vi "控制VI的显示方式.vi"() -> ()   [LabVIEW 2011]
panel:
  in  "方式":T1(ring)
  in  "stop":bool
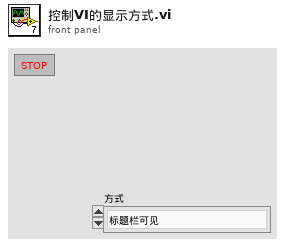
[diagram p1: front panel]
types:
  T1 = enum16{"标题栏可见", "标题栏不可见", "工具栏可见", "工具栏不可见", "菜单条可见", "菜单条不可见"}
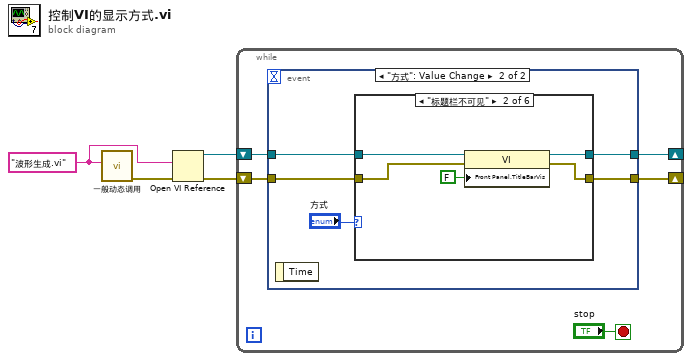
[diagram p0: block diagram]
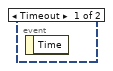
[diagram p2: hidden frame]
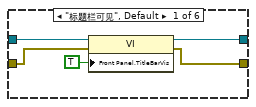
[diagram p3: hidden frame]
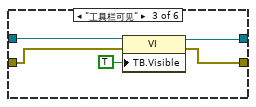
[diagram p4: hidden frame]
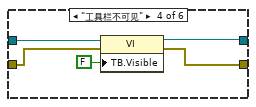
[diagram p5: hidden frame]
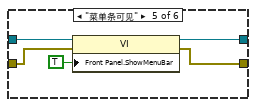
[diagram p6: hidden frame]
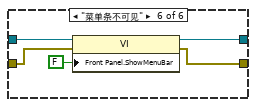
[diagram p7: hidden frame]
diagram:
  w3 = "波形生成.vi" ("name or relative path")
  n1 = call "一般动态调用.vi"("name or relative path"=w3) -> ("error out"=w4:errorcluster)  [unwired: 10 in]
  n2 = Open VI Reference(vi path=w3, error in (no error)=w4) -> (vi reference=w2:refnum<vi>, error out=w1:errorcluster)  [unwired: 4 in]
  n3 = while {
    shift-right: [w6] -> _
    shift-left: w2 -> [w8]
    shift-right: [w5] -> _
    shift-left: w1 -> [w7]
    stop <- "stop" stop-if-true
    n4 = event shown="[1] \"方式\": Value Change" {
      selector: _ -> [_ _]
      dyn-events: _ -> [_ _]
      timeout: _ -> [_ _]
      tunnel: w8 -> [_ w13]
      tunnel: w7 -> [_ w12]
      tunnel: [_ w11] -> w6
      tunnel: [_ w10] -> w5
      event Timeout {
        n5 = event-data() -> ()  [unwired: 1 in, 1 out]
      }
      event "方式": Value Change {
        n6 = event-data() -> ()  [unwired: 1 in, 1 out]
        n7 = case shown="\"标题栏不可见\"" "方式" {
          tunnel: w13 -> [w19 w24 w29 w34 w39 w44]
          tunnel: w12 -> [w18 w23 w28 w33 w38 w43]
          tunnel: [w17 w22 w27 w32 w36 w42] -> w11
          tunnel: [w16 w21 w26 w31 w37 w41] -> w10
          frame "标题栏可见", Default {
            n8 = property class="VI"(reference=w19, error in=w18, "Front Panel.TitleBarVis"=TRUE ("Front Panel Window:Title Bar Visible")) -> (reference out=w17:refnum<vi>, error out=w16:errorcluster)
          }
          frame "标题栏不可见" {
            n9 = property class="VI"(reference=w24, error in=w23, "Front Panel.TitleBarVis"=FALSE ("Front Panel Window:Title Bar Visible")) -> (reference out=w22:refnum<vi>, error out=w21:errorcluster)
          }
          frame "工具栏可见" {
            n10 = property class="VI"(reference=w29, error in=w28, "TB.Visible"=TRUE ("Tool Bar:Visible")) -> (reference out=w27:refnum<vi>, error out=w26:errorcluster)
          }
          frame "工具栏不可见" {
            n11 = property class="VI"(reference=w34, error in=w33, "TB.Visible"=FALSE ("Tool Bar:Visible")) -> (reference out=w32:refnum<vi>, error out=w31:errorcluster)
          }
          frame "菜单条可见" {
            n12 = property class="VI"(reference=w39, error in=w38, "Front Panel.ShowMenuBar"=TRUE ("Front Panel Window:Show Menu Bar")) -> (reference out=w36:refnum<vi>, error out=w37:errorcluster)
          }
          frame "菜单条不可见" {
            n13 = property class="VI"(reference=w44, error in=w43, "Front Panel.ShowMenuBar"=FALSE ("Front Panel Window:Show Menu Bar")) -> (reference out=w42:refnum<vi>, error out=w41:errorcluster)
          }
        }
      }
    }
  }
